vi "Force-Distance curve with offset compensation.vi"() -> ()   [LabVIEW 2016]
doc: "This example perfoms Force-distance measurement with offset compensation.\nIt requires the PLL module to run.\n\n- Nanonis Programming Interface -"
uses:
  Nanonis Prog Interface.lvlib
panel:
  in  "Wait (ms)":u32=50
  in  "Machine name":string="localhost"
  out "Ready":bool
  out "Restore Z-Controller state":bool
  out "Measure force-distance curve":bool
  out "Compensate frequency offet":bool
  out "Wait":bool
  out "Zcont OFF + TipLift":bool caption="Switch Z-Controller OFF + TipLift"
  in  "Tip Lift (m)":sgl format="%_4p"
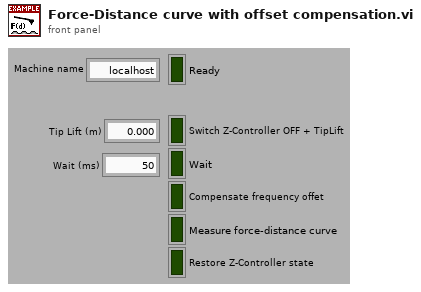
[diagram p1: front panel]
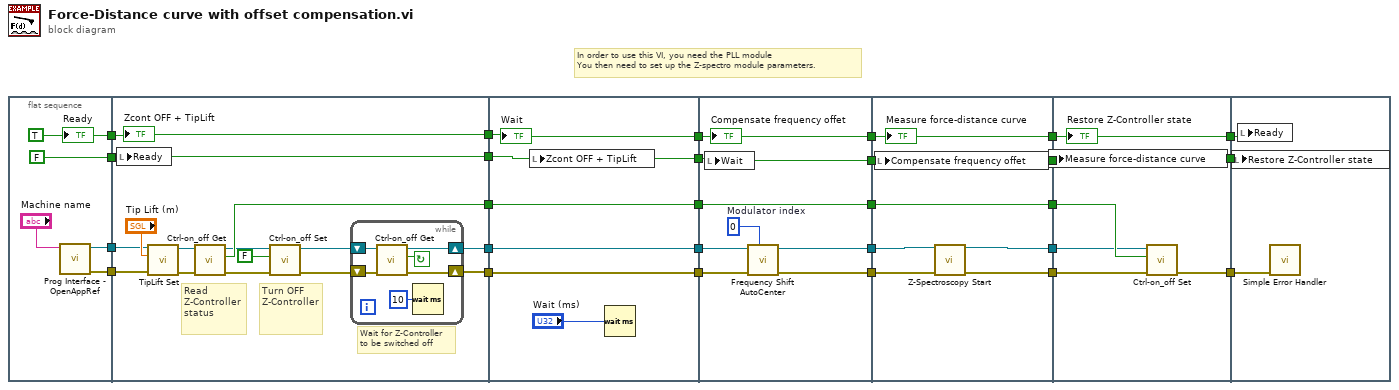
[diagram p0: block diagram]
diagram:
  # "In order to use this VI, you need the PLL module\nYou then need to set up the Z-spectro module parameters."
  n1 = flat-sequence {
    tunnel: [w32] -> w27
    tunnel: [FALSE ("ready")] -> w26
    tunnel: [w30] -> w6
    tunnel: [w28] -> w5
    tunnel: w27 -> [w45]
    tunnel: w26 -> [w44]
    tunnel: [w45] -> w25
    tunnel: [w44] -> w24
    tunnel: [w38] -> w23
    tunnel: [w41] -> w8
    tunnel: w6 -> [w40]
    tunnel: w5 -> [w37]
    tunnel: [w33] -> w3
    tunnel: w25 -> [w59]
    tunnel: w24 -> [w57]
    tunnel: [w59] -> w22
    tunnel: [w57] -> w21
    tunnel: [w56] -> w20
    tunnel: w23 -> [w56]
    tunnel: [w55] -> w9
    tunnel: w8 -> [w55]
    tunnel: [w54] -> w4
    tunnel: w3 -> [w54]
    tunnel: w22 -> [w66]
    tunnel: w21 -> [w65]
    tunnel: w20 -> [w67]
    tunnel: [w66] -> w19
    tunnel: [w65] -> w18
    tunnel: [w64] -> w15
    tunnel: [w63] -> w10
    tunnel: w9 -> [w63]
    tunnel: w4 -> [w62]
    tunnel: [w61] -> w2
    tunnel: w19 -> [w74]
    tunnel: w18 -> [w73]
    tunnel: [w74] -> w17
    tunnel: [w73] -> w16
    tunnel: w15 -> [w72]
    tunnel: [w71] -> w14
    tunnel: [w70] -> w11
    tunnel: w10 -> [w70]
    tunnel: w2 -> [w69]
    tunnel: [w68] -> w1
    tunnel: w17 -> [w79]
    tunnel: w16 -> [w78]
    tunnel: w14 -> [w80]
    tunnel: [w79] -> w13
    tunnel: [w78] -> w12
    tunnel: w11 -> [w77]
    tunnel: [w76] -> w7
    tunnel: w1 -> [w75]
    tunnel: w13 -> [w83]
    tunnel: w12 -> [w82]
    tunnel: w7 -> [w81]
    frame #0 {
      w32 = TRUE ("ready")
      n2 = call <userlib>:"Prog Interface - OpenAppRef.vi"("Machine name (local machine IP)"="Machine name") -> ("Error out"=w30:errorcluster, "Application reference"=w28:refnum<vi>)  [unwired: 5 in]
      "Ready" <- w32
    }
    frame #1 {
      # "Turn OFF \nZ-Controller"
      # "Read \nZ-Controller\nstatus"
      # "Wait for Z-Controller\nto be switched off"
      n3 = local write "Ready"(w44) -> ()
      n4 = call <userlib>:"TipLift Set.vi"("error in (no error)"=w40, "TipLift (m)"="Tip Lift (m)", "Application ref in"=w37) -> ("error out"=w43:errorcluster, "Application ref out"=w36:refnum<vi>)  [unwired: 7 in]
      n5 = call <userlib>:"Ctrl-on_off Get.vi"("error in (no error)"=w43, "Application ref in"=w36) -> ("error out"=w42:errorcluster, "Z-Controller on/off status"=w41:bool, "Application ref out"=w35:refnum<vi>)  [unwired: 7 in]
      n6 = call <userlib>:"Ctrl-on_off Set.vi"("error in (no error)"=w42, "Z Controller ON/OFF"=FALSE ("Ctrl on/off"), "Application ref in"=w35) -> ("error out"=w39:errorcluster, "Application ref out"=w34:refnum<vi>)  [unwired: 7 in]
      n7 = while {
        shift-right: [w53] -> w38
        shift-left: w39 -> [w52]
        shift-right: [w48] -> w33
        shift-left: w34 -> [w49]
        stop <- w51 continue-if-true
        n8 = call <userlib>:"Ctrl-on_off Get.vi"("error in (no error)"=w52, "Application ref in"=w49) -> ("error out"=w53:errorcluster, "Z-Controller on/off status"=w51:bool, "Application ref out"=w48:refnum<vi>)  [unwired: 7 in]
        n9 = Wait (ms)(milliseconds to wait=u32 10) -> ()  [unwired: 1 out]
      }
      "Zcont OFF + TipLift" <- w45
    }
    frame #2 {
      n10 = local write "Zcont OFF + TipLift"(w57) -> ()
      n11 = Wait (ms)(milliseconds to wait="Wait (ms)") -> ()  [unwired: 1 out]
      "Wait" <- w59
    }
    frame #3 {
      w60 = 0  # Modulator index
      n12 = local write "Wait"(w65) -> ()
      n13 = call <userlib>:"Frequency Shift AutoCenter.vi"("Modulator index"=w60, "Error in (no error)"=w67, "Application ref in"=w62) -> ("Error out"=w64:errorcluster, "Application ref out"=w61:refnum<vi>)  [unwired: 7 in]
      "Compensate frequency offet" <- w66
    }
    frame #4 {
      n14 = local write "Compensate frequency offet"(w73) -> ()
      n15 = call <userlib>:"Z-Spectroscopy Start.vi"("Application ref in"=w69, "error in (no error)"=w72) -> ("Application ref out"=w68:refnum<vi>, "error out"=w71:errorcluster)  [unwired: 9 in, 3 out]
      "Measure force-distance curve" <- w74
    }
    frame #5 {
      n16 = local write "Measure force-distance curve"(w78) -> ()
      n17 = call <userlib>:"Ctrl-on_off Set.vi"("error in (no error)"=w80, "Z Controller ON/OFF"=w77, "Application ref in"=w75) -> ("error out"=w76:errorcluster)  [unwired: 7 in, 1 out]
      "Restore Z-Controller state" <- w79
    }
    frame #6 {
      n18 = local write "Restore Z-Controller state"(w82) -> ()
      n19 = local write "Ready"(w83) -> ()
      n20 = call <vilib>:"Simple Error Handler.vi"("error in (no error)"=w81) -> ()  [unwired: 4 in, 5 out]
    }
  }
